vi "Init.vi"(8 "error in (no error)":errorcluster, 10 "JSON":string, 11 "Type":string) -> (0 "error out":errorcluster, 3 "JSONRequest out":refnum<class "JSONRequest.lvclass">)   [LabVIEW 2020, in "obs-websocket.lvlib" / "JSONRequest.lvclass"]
uses:
  JSONRequest.lvclass
  JSONRequest.lvclass/JSONRequest.ctl
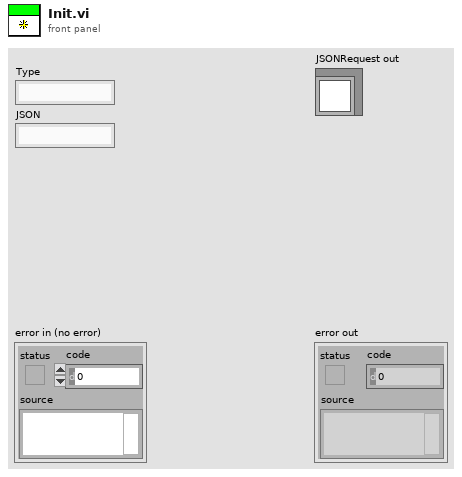
[diagram p1: front panel]
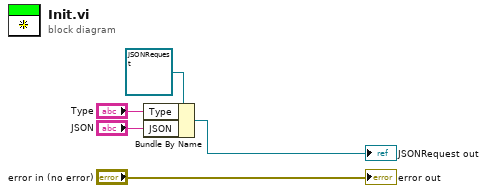
[diagram p0: block diagram]
diagram:
  n1 = Bundle By Name(cluster=refnum<class "JSONRequest.lvclass"> refnum ("JSONRequest in"), "Type"="Type", "JSON"="JSON") -> (→"JSONRequest out":refnum<class "JSONRequest.lvclass">)
  "error out" <- "error in (no error)"
